vi "Test Valid Multiple Channels Registration.vi"() -> ()   [LabVIEW 2024]
uses:
  Mock Sift Proxy Server/Mock Sift Proxy Server.lvclass
  Sift API/Sift Client.lvclass
  Sift API/Types/Data Type.ctl
  Sift Client.lvlib
panel:
  out "Server Error":errorcluster
  out "Success 2":bool
  out "Error 2":errorcluster
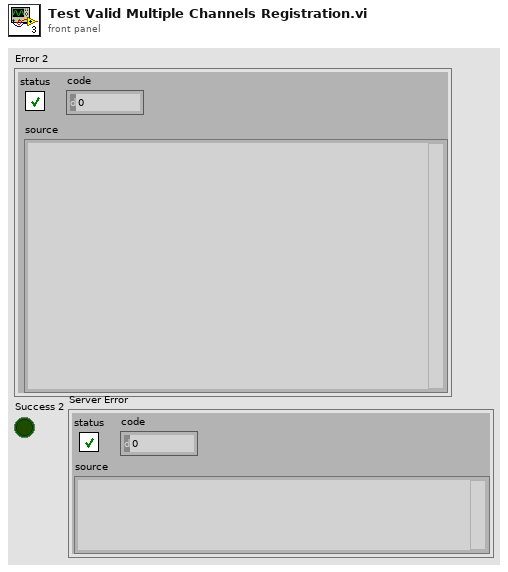
[diagram p1: front panel]
types:
  T1 = typedef "Sift Client.lvlib/Data Type.ctl" = enum8{"double", "float", "uint64", "int64", "uint32", "int32", "bool", "bit field", "enum"}
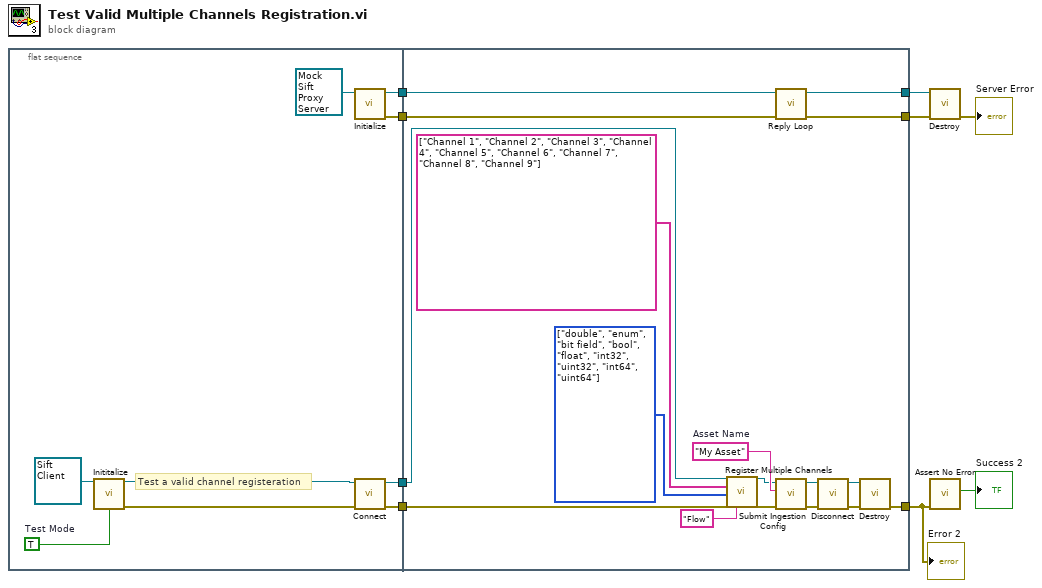
[diagram p0: block diagram]
diagram:
  n1 = flat-sequence {
    tunnel: [w17] -> w9
    tunnel: [w12] -> w8
    tunnel: [w11] -> w7
    tunnel: [w10] -> w6
    tunnel: [w30] -> w5
    tunnel: w9 -> [w31]
    tunnel: [w34] -> w1
    tunnel: w8 -> [w29]
    tunnel: w7 -> [w28]
    tunnel: w6 -> [w25]
    tunnel: [w24] -> w4
    frame #0 {
      w15 = TRUE  # Test Mode
      # "Test a valid channel registeration"
      n2 = call-dynamic "Inititalize.vi"("Sift Client in"=refnum<class "Sift Client.lvclass"> refnum ("Sift Client.lvlib:Sift Client.lvclass"), "Test Mode"=w15) -> ("Sift Client out"=w13:refnum<class "Sift Client.lvclass">, "error out"=w14:errorcluster)  [unwired: 12 in]
      n3 = call-dynamic "Initialize.vi"("Mock Sift Proxy Server in"=refnum<class "Mock Sift Proxy Server.lvclass"> refnum ("Mock Sift Proxy Server.lvclass")) -> ("error out"=w10:errorcluster, "Mock Sift Proxy Server out"=w17:refnum<class "Mock Sift Proxy Server.lvclass">)  [unwired: 9 in]
      n4 = call-dynamic "Connect.vi"("error in (no error)"=w14, "Sift Client in"=w13) -> ("error out"=w12:errorcluster, "Sift Client out"=w11:refnum<class "Sift Client.lvclass">)  [unwired: 7 in, 1 out]
    }
    frame #1 {
      w19 = T1[] [enum."double", enum."enum", enum."bit field", enum."bool", enum."float", enum."int32", enum."uint32", enum."int64", enum."uint64"] items=["double", "float", "uint64", "int64", "uint32", "int32", "bool", "bit field", "enum"]
      w33 = "My Asset"  # Asset Name
      n5 = call "Register Multiple Channels.vi"("Sift Client in"=w28, "Names"=string[] ["Channel 1", "Channel 2", "Channel 3", "Channel 4", "Channel 5", "Channel 6", "Channel 7", "Channel 8", "Channel 9"], "Data Types"=w19, "error in (no error)"=w29, "Flow Name"="Flow") -> ("Sift Client out"=w32:refnum<class "Sift Client.lvclass">, "error out"=w35:errorcluster)  [unwired: 21 in]
      n6 = call-dynamic "Reply Loop.vi"("error in (no error)"=w25, "Mock Sift Proxy Server in"=w31) -> ("error out"=w24:errorcluster, "Mock Sift Proxy Server out"=w30:refnum<class "Mock Sift Proxy Server.lvclass">)  [unwired: 8 in]
      n7 = call-dynamic "Submit Ingestion Config.vi"("error in (no error)"=w35, "Asset Name"=w33, "Sift Client in"=w32) -> ("error out"=w21:errorcluster, "Sift Client out"=w22:refnum<class "Sift Client.lvclass">)  [unwired: 7 in]
      n8 = call-dynamic "Disconnect.vi"("error in (no error)"=w21, "Sift Client in"=w22) -> ("error out"=w26:errorcluster, "Sift Client out"=w27:refnum<class "Sift Client.lvclass">)  [unwired: 8 in]
      n9 = call-dynamic "Destroy.vi"("error in (no error)"=w26, "Sift Client in"=w27) -> ("error out"=w34:errorcluster)  [unwired: 8 in, 1 out]
    }
  }
  n10 = call-dynamic "Destroy.vi"("error in (no error)"=w4, "Mock Sift Proxy Server in"=w5) -> ("error out"=→"Server Error":errorcluster)  [unwired: 8 in, 1 out]
  n11 = call "Assert No Error.vi"("Error"=w1) -> ("Success"=→"Success 2":bool)  [unwired: 10 in]
  "Error 2" <- w1
